vi "Is Valid Number (SGL 2D Array).vi"(2 "SGL 2D Array":sgl[][](array[numeric])) -> (7 "Is Valid Number? (2D)":bool[][](array[boolean]))   [LabVIEW 2021, in "Comparison.lvlib"]
uses:
  Is a Valid Number (SGL).vi
  Comparison.lvlib
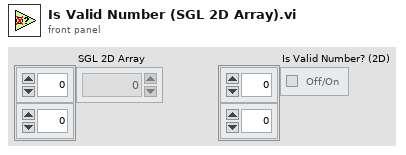
[diagram p1: front panel]
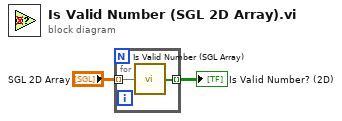
[diagram p0: block diagram]
diagram:
  n1 = for {
    tunnel: [w4] -> w1 mode=indexing
    tunnel: "SGL 2D Array" -> [w3] mode=indexing
    n2 = call "Is Valid Number (SGL Array).vi"("SGL Array"=w3) -> ("Is Valid Number? (1D)"=w4:bool[])  [unwired: 8 in]
  }
  "Is Valid Number? (2D)" <- w1
